vi "Telescope get object reference.vi"(8 "error in (no error)":errorcluster, 11 "Telescope Name":string) -> (0 "error out":errorcluster, 2 "Telescope Name dup":string, 3 "PRIME Telescope.lvclass":refnum<class "Telescope.lvclass">)   [LabVIEW 2024]
uses:
  Telescope.lvclass
  Telescope Simulator/Telescope Simulator.lvclass
  PRIME Telescope/PRIME Telescope.lvclass
  LDT Telescope/LDT Telescope.lvclass
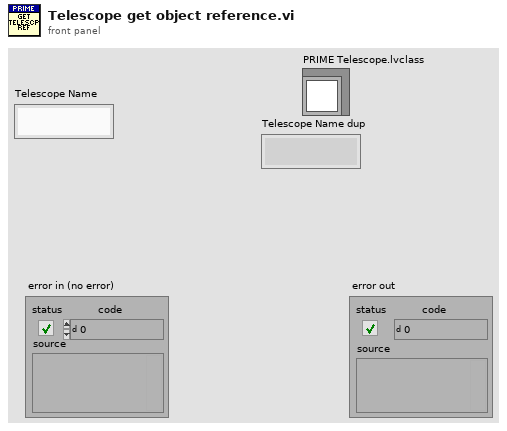
[diagram p1: front panel]
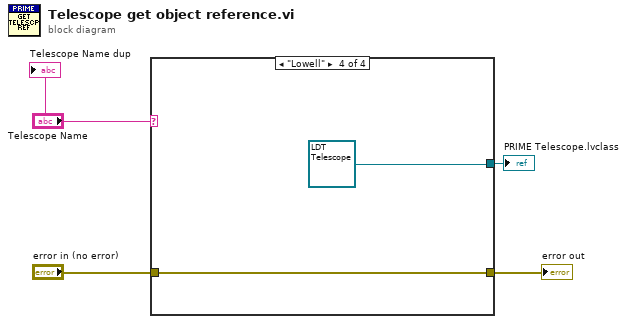
[diagram p0: block diagram]
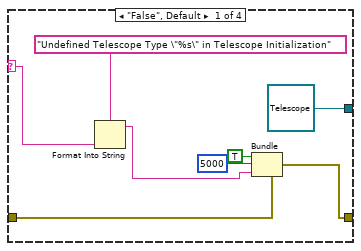
[diagram p2: hidden frame]
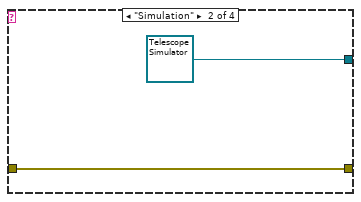
[diagram p3: hidden frame]
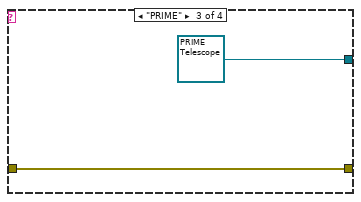
[diagram p4: hidden frame]
diagram:
  n1 = case shown="\"Lowell\"" "Telescope Name" {
    selector: "Telescope Name" -> [w7 _ _ _]
    tunnel: [refnum<class "Telescope.lvclass"> refnum ("Telescope.lvclass") refnum<class "Telescope Simulator.lvclass"> refnum ("Telescope Simulator.lvclass") refnum<class "PRIME Telescope.lvclass"> refnum ("PRIME Telescope.lvclass") refnum<class "LDT Telescope.lvclass"> refnum ("LDT Telescope.lvclass")] -> w1
    tunnel: "error in (no error)" -> [w12 w13 w15 w17]
    tunnel: [w5 w13 w15 w17] -> w2
    frame "False", Default {
      n2 = Format Into String(format string="Undefined Telescope Type \"%s\" in Telescope Initialization", w7) -> (resulting string=w6:string)  [unwired: 2 in, 1 out]
      n3 = Bundle(cluster=w12, "status"=TRUE, "code"=5000, "source"=w6) -> (w5:errorcluster)
    }
    frame "Simulation" {
    }
    frame "PRIME" {
    }
    frame "Lowell" {
    }
  }
  "error out" <- w2
  "PRIME Telescope.lvclass" <- w1
  "Telescope Name dup" <- "Telescope Name"
